vi "Actor Core.vi"(8 "error in":cluster{"状态":bool, "代码":i32, "源":string} caption="错误输入", 11 "仿真蒸发冷却器":refnum<class "Simulated Evaporative Cooler.lvclass">) -> (0 "error out":cluster{"状态":bool, "代码":i32, "源":string} caption="错误输出", 3 "操作者输出":refnum<class "Actor.lvclass">)   [LabVIEW 2013, in "Simulated Evaporative Cooler.lvclass"]
doc: "Actor Core.vi包含操作者的主要消息处理循环。操作者通常位于该循环中，在各种消息到达时对消息进行处理。如Do.vi消息返回任何错误，该循环将停止运行，错误代码43将被作为“无错误停止”的标准信号发送给调用方。如需更改上述行为，可在子孙类的Handle Error.vi中对该部分逻辑进行重写。"
uses:
  Simulated Evaporative Cooler.lvclass
  <vilib>/ActorFramework/Actor/Actor.lvclass
  Evaporative Cooler/Evaporative Cooler/Evaporative Cooler.lvclass
  Simulation Data_Global.vi
panel:
  out "停止信号":bool
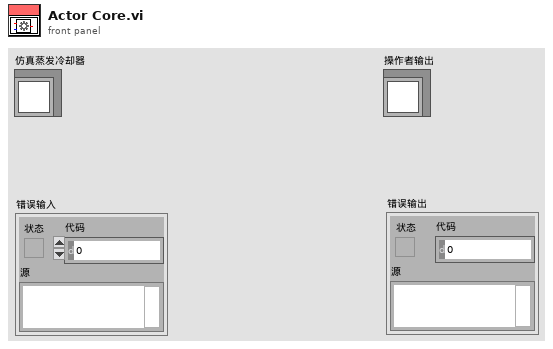
[diagram p1: front panel]
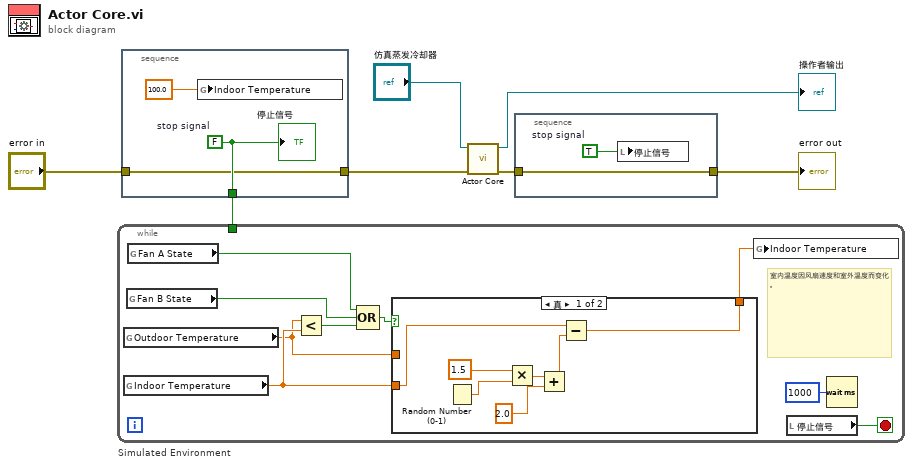
[diagram p0: block diagram]
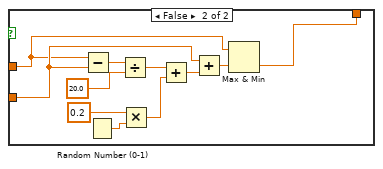
[diagram p2: hidden frame]
diagram:
  n1 = stacked-sequence {
    tunnel: [w10] -> w7
    tunnel: [w9] -> w4
    tunnel: "error in" -> [w9]
    frame #0 {
      w10 = FALSE  # stop signal
      n2 = global write "Simulation Data_Global.vi" "Indoor Temperature"(100.0 ("Temperature")) -> ()
      "停止信号" <- w10
    }
  }
  n3 = while "Simulated Environment" {
    tunnel: w7 -> [_]
    stop <- w18 stop-if-true
    # "室内温度因风扇速度和室外温度而变化。"
    n4 = global read "Simulation Data_Global.vi" "Outdoor Temperature"() -> (w14:dbl)
    n5 = global read "Simulation Data_Global.vi" "Indoor Temperature"() -> (w15:dbl)
    n6 = global read "Simulation Data_Global.vi" "Fan B State"() -> (w12:bool)
    n7 = global read "Simulation Data_Global.vi" "Fan A State"() -> (w13:bool)
    n8 = Less?(x=w14, y=w15) -> (x < y?=w16:bool)
    n9 = Compound Arithmetic op=OR(w13, w12, w16) -> (w19:bool)
    n10 = case shown="真" w19 {
      tunnel: w15 -> [w21 w29]
      tunnel: w14 -> [_ w28]
      tunnel: [w20 w27] -> w11
      frame True {
        n11 = Random Number (0-1)() -> (number: 0 to 1=w25:dbl)
        n12 = Multiply(x=1.5 ("y"), y=w25) -> (x*y=w24:dbl)
        n13 = Add(x=w24, y=2.0) -> (x+y=w22:dbl)
        n14 = Subtract(x=w21, y=w22) -> (x-y=w20:dbl)
      }
      frame False {
        n15 = Subtract(x=w28, y=w29) -> (x-y=w37:dbl)
        n16 = Random Number (0-1)() -> (number: 0 to 1=w33:dbl)
        n17 = Divide(x=w37, y=20.0) -> (x/y=w35:dbl)
        n18 = Multiply(x=0.2, y=w33) -> (x*y=w32:dbl)
        n19 = Add(x=w35, y=w32) -> (x+y=w31:dbl)
        n20 = Add(x=w29, y=w31) -> (x+y=w30:dbl)
        n21 = Max & Min(x=w28, y=w30) -> (min(x,y)=w27:dbl)  [unwired: 1 out]
      }
    }
    n22 = global write "Simulation Data_Global.vi" "Indoor Temperature"(w11) -> ()
    n23 = local read "停止信号"() -> (w18:bool)
    n24 = Wait (ms)(milliseconds to wait=u32 1000) -> ()  [unwired: 1 out]
  }
  n25 = call-parent "Actor Core.vi"("error in"=w4, "蒸发冷却器"="仿真蒸发冷却器") -> ("error out"=w1:cluster{"状态":bool, "代码":i32, "源":string}, "操作者输出"=→"操作者输出":refnum<class "Actor.lvclass">)  [unwired: 8 in]
  n26 = stacked-sequence {
    tunnel: [w38] -> w2
    tunnel: w1 -> [w38]
    frame #0 {
      w39 = TRUE  # stop signal
      n27 = local write "停止信号"(w39) -> ()
    }
  }
  "error out" <- w2
